vi "Register for Car Wash Model Notification Messages.vi"(8 "error in (no error)":errorcluster, 11 "Car Wash Model in":refnum<class "Car Wash Model.lvclass">) -> (0 "error out":errorcluster, 3 "Car Wash Model out":refnum<class "Car Wash Model.lvclass">)   [LabVIEW 2019, in "Car Wash Model.lvclass"]
uses:
  <vilib>/gpm_packages/@cs/Car-wash/Source/Car Wash Model/Car Wash Model/Car Wash Model.lvclass
  C:/Program Files/National Instruments/LabVIEW 2019/vi.lib/gpm_packages/@cs/mva-core/Source/IObserver/IObserver/IObserver.lvclass
  <vilib>/gpm_packages/@cs/Car-wash/Source/Car Wash Model/Car Wash Model Messages/Start Car Wash Msg/Start Car Wash Msg.lvclass
  C:/Program Files/National Instruments/LabVIEW 2019/vi.lib/gpm_packages/@cs/transport/Source/Concrete/ActorMessageTransport/Notification Msg/Notification Msg.lvclass
  <vilib>/gpm_packages/@cs/Car-wash/Source/Car Wash Model/Car Wash Model Messages/Handle Vehicle out of Position Msg/Handle Vehicle out of Position Msg.lvclass
  <vilib>/gpm_packages/@cs/Car-wash/Source/Car Wash Model/Car Wash Model Messages/Stop Car Wash Msg/Stop Car Wash Msg.lvclass
  <vilib>/gpm_packages/@cs/Car-wash/Source/Car Wash Model/Car Wash Model Messages/Start Batch Car Wash Msg/Start Batch Car Wash Msg.lvclass
  <vilib>/gpm_packages/@cs/mva-core/Source/SubscriptionPolicy/BasicSubscription/BasicSubscription.lvclass/BasicSubscription.ctl
  <vilib>/ActorFramework/Actor/Actor.lvclass/Actor.ctl
  <vilib>/ActorFramework/Message Enqueuer/Message Enqueuer.lvclass/Message Enqueuer.ctl
  <vilib>/gpm_packages/@cs/transport/Source/Concrete/ActorMessageTransport/ActorMessageTransport.lvclass/ActorMessageTransport.ctl
  <vilib>/gpm_packages/@cs/mva-core/Source/IMediator/SubscriptionRequest/SubscriptionRequest.lvclass/SubscriptionRequest.ctl
  <vilib>/gpm_packages/@cs/mva-core/Source/IObserver/IObserver Messages/Subscribe Msg/Subscribe Msg.lvclass/Subscribe Msg.ctl
  <vilib>/gpm_packages/@cs/Car-wash/Source/Car Wash Model/Car Wash Model/Car Wash Model.lvclass/Car Wash Model.ctl
  <vilib>/gpm_packages/@cs/mva-core/Source/IMediator/SubscriptionRequest/Pack Subscription Request.vi
  <vilib>/gpm_packages/@cs/mva-core/Source/IObserver/IObserver Messages/Subscribe Msg/Send Subscribe.vi
  <vilib>/ActorFramework/Actor/Read Self Enqueuer.vi
  <vilib>/gpm_packages/@cs/transport/Source/Concrete/ActorMessageTransport/Construct Actor Message Transport.vi
  <vilib>/ActorFramework/Message Enqueuer/Enqueue.vi
  <vilib>/ActorFramework/Message Enqueuer/Init from Existing Queue.vi
  <vilib>/ActorFramework/Message Enqueuer/Equals Not A Refnum.vi
  <vilib>/gpm_packages/@cs/mva-core/Source/SubscriptionPolicy/BasicSubscription/BasicSubscription.lvclass
  C:/Program Files/National Instruments/LabVIEW 2019/vi.lib/gpm_packages/@cs/mva-core/Source/IMediator/ISubscriptionPolicy/ISubscriptionPolicy.lvclass
  <vilib>/gpm_packages/@cs/mva-core/Source/IObserver/IObserver/IObserver.lvclass
  C:/Program Files/National Instruments/LabVIEW 2019/vi.lib/ActorFramework/Actor/Actor.lvclass
  <vilib>/gpm_packages/@cs/transport/Source/Concrete/ActorMessageTransport/ActorMessageTransport.lvclass
  C:/Program Files/National Instruments/LabVIEW 2019/vi.lib/gpm_packages/@cs/transport/Source/ITransport/ITransport.lvclass
  <vilib>/gpm_packages/@cs/mva-core/Source/IObserver/IObserver Messages/Subscribe Msg/Subscribe Msg.lvclass
  C:/Program Files/National Instruments/LabVIEW 2019/vi.lib/ActorFramework/Message/Message.lvclass
  <vilib>/Utility/error.llb/Error Cluster From Error Code.vi
  <vilib>/gpm_packages/@cs/mva-core/Source/IMediator/ISubscriptionPolicy/Open Subscription Policy.vi
  <vilib>/ActorFramework/Message Priority Queue/Priority Enqueue.vi
  <vilib>/ActorFramework/Message Enqueuer/Message Enqueuer.lvclass
  <vilib>/gpm_packages/@cs/mva-core/Source/IMediator/SubscriptionRequest/SubscriptionRequest.lvclass
  <vilib>/gpm_packages/@cs/transport/Source/Concrete/ActorMessageTransport/Notification Msg/Notification Msg.lvclass
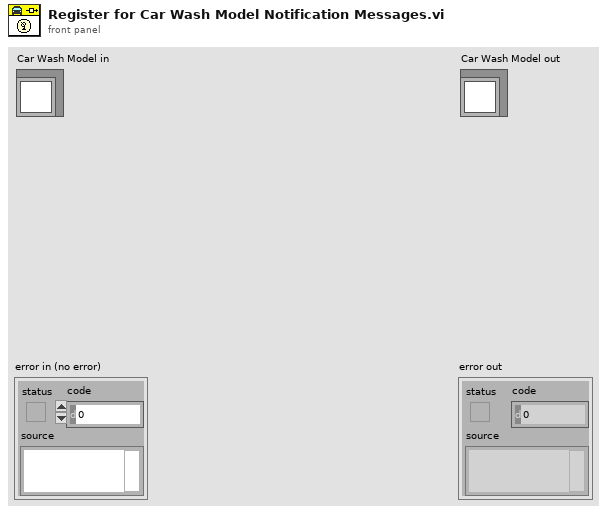
[diagram p1: front panel]
types:
  T1 = typedef "IMediator.lvlib/ISubscriptionPolicy.lvclass/ISubscriptionPolicy Reference.ctl" = refnum<data-value>
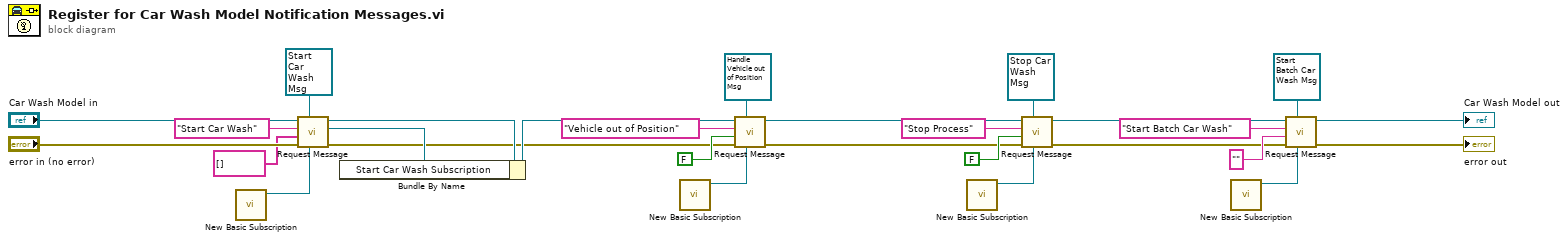
[diagram p0: block diagram]
diagram:
  n1 = call <vilib>:"New Basic Subscription.vi"() -> ("BasicSubscription Out"=w23:refnum<class "BasicSubscription.lvclass">)  [unwired: 11 in]
  n2 = call <vilib>:"Request Message.vi"("Configured SubscriptionPolicy"=w23, "Desired Notification Msg"=refnum<class "Start Car Wash Msg.lvclass"> refnum ("Start Car Wash Msg.lvclass"), "error in (no error)"="error in (no error)", "Data Type"=string[] [], "Datum Name"="Start Car Wash", "IObserver in"="Car Wash Model in") -> ("error out"=w15:errorcluster, "Subscription Policy"=w21:T1, "IObserver out"=w22:refnum<class "Car Wash Model.lvclass">)  [unwired: 3 in]
  n3 = Bundle By Name(cluster=w22, "Start Car Wash Subscription"=w21) -> (w16:refnum<class "Car Wash Model.lvclass">)
  n4 = call <vilib>:"New Basic Subscription.vi"() -> ("BasicSubscription Out"=w18:refnum<class "BasicSubscription.lvclass">)  [unwired: 11 in]
  n5 = call <vilib>:"Request Message.vi"("Configured SubscriptionPolicy"=w18, "Desired Notification Msg"=refnum<class "Handle Vehicle out of Position Msg.lvclass"> refnum ("Handle Vehicle out of Position Msg.lvclass"), "error in (no error)"=w15, "Data Type"=FALSE, "Datum Name"="Vehicle out of Position", "IObserver in"=w16) -> ("error out"=w10:errorcluster, "IObserver out"=w11:refnum<class "Car Wash Model.lvclass">)  [unwired: 3 in, 1 out]
  n6 = call <vilib>:"New Basic Subscription.vi"() -> ("BasicSubscription Out"=w14:refnum<class "BasicSubscription.lvclass">)  [unwired: 11 in]
  n7 = call <vilib>:"Request Message.vi"("Configured SubscriptionPolicy"=w14, "Desired Notification Msg"=refnum<class "Stop Car Wash Msg.lvclass"> refnum ("Stop Car Wash Msg.lvclass"), "error in (no error)"=w10, "Data Type"=FALSE, "Datum Name"="Stop Process", "IObserver in"=w11) -> ("error out"=w3:errorcluster, "IObserver out"=w5:refnum<class "Car Wash Model.lvclass">)  [unwired: 3 in, 1 out]
  n8 = call <vilib>:"New Basic Subscription.vi"() -> ("BasicSubscription Out"=w6:refnum<class "BasicSubscription.lvclass">)  [unwired: 11 in]
  n9 = call <vilib>:"Request Message.vi"("Configured SubscriptionPolicy"=w6, "Desired Notification Msg"=refnum<class "Start Batch Car Wash Msg.lvclass"> refnum ("Start Batch Car Wash Msg.lvclass"), "error in (no error)"=w3, "Data Type"="", "Datum Name"="Start Batch Car Wash", "IObserver in"=w5) -> ("error out"=→"error out":errorcluster, "IObserver out"=→"Car Wash Model out":refnum<class "Car Wash Model.lvclass">)  [unwired: 3 in, 1 out]
